vi "SW_Gen_Get_Bounding_rectangles_DAQmx.vi"(2 "Width of the borders combined":cluster{"Width":i32, "Height":i32}, 3 "Draw Area Size":T3, 4 "Image geometrical and scaling parameters":T2) -> (1 "Bounding rectangles":T1)   [LabVIEW 2018, in "Tracker.lvlib"]
uses:
  Tracker.lvlib
  Controls/CTL_Draw_Area_Size.ctl
  Controls/CTL_Image_Geometrical_and_scaling_parameters.ctl
  Controls/CTL_Bounding_Rectangle_of_Segments.ctl
  Common_Resources.lvlib
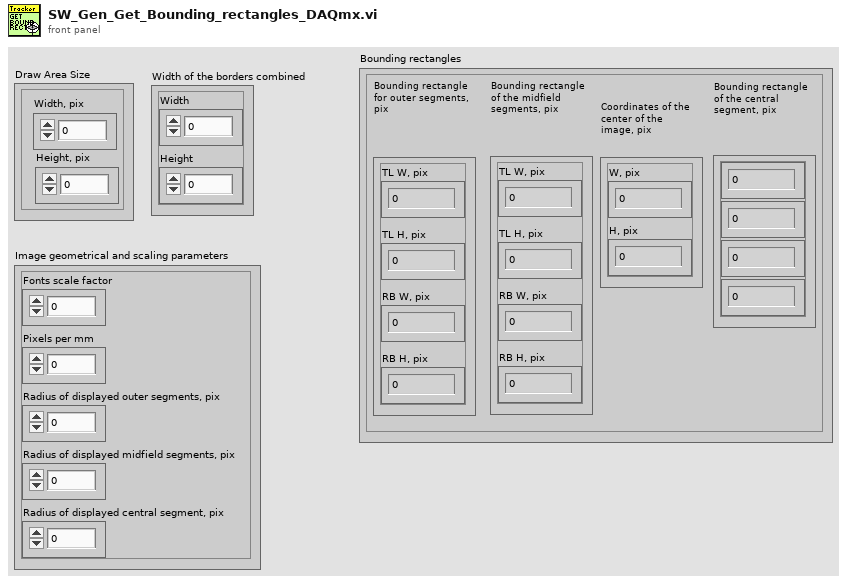
[diagram p1: front panel]
types:
  T1 = typedef "Common_Resources.lvlib/CTL_Bounding_Rectangle_of_Segments.ctl" = cluster{"Bounding rectangle for outer segments, pix":cluster{"TL W, pix":i32, "TL H, pix":i32, "RB W, pix":i32, "RB H, pix":i32}, "Bounding rectangle of the midfield segments, pix":cluster{"TL W, pix":i32, "TL H, pix":i32, "RB W, pix":i32, "RB H, pix":i32}, "Coordinates of the center of the image, pix":cluster{"W, pix":i32, "H, pix":i32}, "Bounding rectangle of the central segment, pix":cluster{"Numeric Control":i32, "Numeric Control":i32, "Numeric Control":i32, "Numeric Control":i32}}
  T2 = typedef "Common_Resources.lvlib/CTL_Image_Geometrical_and_scaling_parameters.ctl" = cluster{"Fonts scale factor":dbl, "Pixels per mm":dbl, "Radius of displayed outer segments, pix":dbl, "Radius of displayed midfield segments, pix":dbl, "Radius of displayed central segment, pix":dbl}
  T3 = typedef "Common_Resources.lvlib/CTL_Draw_Area_Size.ctl" = cluster{"Width, pix":i32, "Height, pix":i32}
  T4 = cluster{cluster{dbl, dbl, dbl, dbl}, cluster{dbl, dbl, dbl, dbl}, cluster{dbl, dbl}, cluster{dbl, dbl, dbl, dbl}}
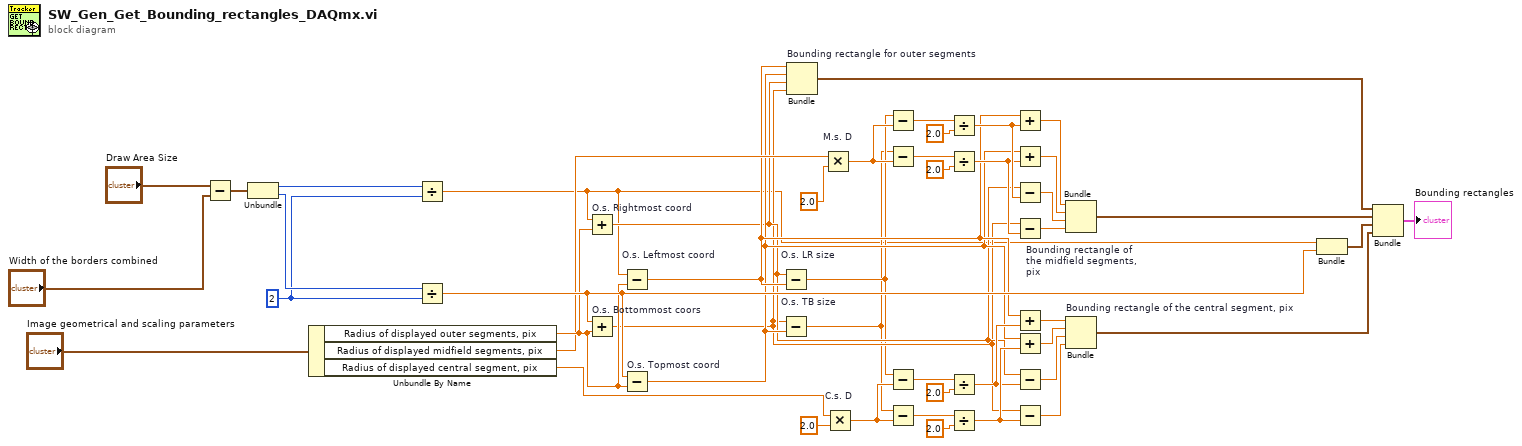
[diagram p0: block diagram]
diagram:
  w42 = u32 2 ("y")
  n1 = Subtract(x="Draw Area Size", y="Width of the borders combined") -> (x-y=w44:T3)
  n2 = Unbundle(w44) -> ("Width, pix"=w46:i32, "Height, pix"=w47:i32)
  n3 = Unbundle By Name("Image geometrical and scaling parameters") -> ("Radius of displayed outer segments, pix"=w23:dbl, "Radius of displayed midfield segments, pix"=w22:dbl, "Radius of displayed central segment, pix"=w2:dbl)
  n4 = Divide(x=w46, y=w42) -> (x/y=w3:dbl)
  n5 = Divide(x=w47, y=w42) -> (x/y=w40:dbl)
  n6 = Add "O.s. Rightmost coord"(x=w3, y=w23) -> (x+y=w7:dbl)
  n7 = Add "O.s. Bottommost coors"(x=w40, y=w23) -> (x+y=w6:dbl)
  n8 = Subtract "O.s. Leftmost coord"(x=w3, y=w23) -> (x-y=w9:dbl)
  n9 = Subtract "O.s. Topmost coord"(x=w40, y=w23) -> (x-y=w8:dbl)
  n10 = Subtract "O.s. LR size"(x=w7, y=w9) -> (x-y=w5:dbl)
  n11 = Subtract "O.s. TB size"(x=w6, y=w8) -> (x-y=w4:dbl)
  n12 = Bundle "Bounding rectangle for outer segments"(w9, w8, w7, w6) -> (w27:cluster{dbl, dbl, dbl, dbl})  [unwired: 1 in]
  n13 = Multiply "M.s. D"(x=w22, y=2.0) -> (x*y=w35:dbl)
  n14 = Multiply "C.s. D"(x=w2, y=2.0) -> (x*y=w14:dbl)
  n15 = Subtract(x=w5, y=w35) -> (x-y=w38:dbl)
  n16 = Subtract(x=w4, y=w35) -> (x-y=w33:dbl)
  n17 = Subtract(x=w5, y=w14) -> (x-y=w11:dbl)
  n18 = Subtract(x=w4, y=w14) -> (x-y=w16:dbl)
  n19 = Divide(x=w38, y=2.0) -> (x/y=w36:dbl)
  n20 = Divide(x=w33, y=2.0) -> (x/y=w32:dbl)
  n21 = Divide(x=w11, y=2.0) -> (x/y=w13:dbl)
  n22 = Divide(x=w16, y=2.0) -> (x/y=w17:dbl)
  n23 = Add(x=w9, y=w36) -> (x+y=w31:dbl)
  n24 = Add(x=w8, y=w32) -> (x+y=w29:dbl)
  n25 = Subtract(x=w7, y=w36) -> (x-y=w30:dbl)
  n26 = Subtract(x=w6, y=w32) -> (x-y=w28:dbl)
  n27 = Add(x=w9, y=w13) -> (x+y=w18:dbl)
  n28 = Add(x=w8, y=w17) -> (x+y=w20:dbl)
  n29 = Subtract(x=w7, y=w13) -> (x-y=w19:dbl)
  n30 = Subtract(x=w6, y=w17) -> (x-y=w21:dbl)
  n31 = Bundle "Bounding rectangle of the midfield segments, pix"(w31, w29, w30, w28) -> (w26:cluster{dbl, dbl, dbl, dbl})  [unwired: 1 in]
  n32 = Bundle "Bounding rectangle of the central segment, pix"(w18, w20, w19, w21) -> (w1:cluster{dbl, dbl, dbl, dbl})  [unwired: 1 in]
  n33 = Bundle ("Coordinates of the center of the image")(w3, w40) -> (w25:cluster{dbl, dbl})  [unwired: 1 in]
  n34 = Bundle(w27, w26, w25, w1) -> (→"Bounding rectangles":T4)  [unwired: 1 in]
